vi "capstone2.vi"() -> ()   [LabVIEW 2016]
uses:
  <instrlib>/Dynamixel Motor/Public/Motor Operation/Low Level/Baud Setting.ctl
  <vilib>/myRIO/Instrument Drivers/Onboard IO/DIO/typedefs/DIO Reference.ctl
  <vilib>/myRIO/Common/Instrument Driver Framework/Utilities/typedefs/myRIO Generic Hardware Reference.ctl
  <vilib>/myRIO/Common/Instrument Driver Framework/Utilities/typedefs/Hardware Version Enum.ctl
  <vilib>/myRIO/Common/Instrument Driver Framework/Utilities/typedefs/myRIO v1.0 Reference.ctl
  <vilib>/myRIO/Common/Instrument Driver Framework/Utilities/typedefs/Generic FPGA Reference.ctl
  <vilib>/myRIO/Common/Instrument Driver Framework/myRIO v1.0/DIO/typedefs/DIO Channels List.ctl
  <vilib>/myRIO/Common/Instrument Driver Framework/myRIO v1.0/DIO/typedefs/DIO Channels Enum.ctl
  <vilib>/userdefined/High Color/nirio_resource_hc.ctl
  <vilib>/myRIO/Common/Instrument Driver Framework/Utilities/vis/Is FPGA Ref Available.vi
  <vilib>/myRIO/Common/Instrument Driver Framework/myRIO v1.0/DIO/vis/myRIO v1.1 Open DIO.vi
  <vilib>/myRIO/Instrument Drivers/Onboard IO/DIO/vis/Write.vi
  <vilib>/myRIO/Common/Instrument Driver Framework/Utilities/vis/Validate Channels.vi
  <vilib>/myRIO/Common/Instrument Driver Framework/myRIO v1.0/DIO/vis/myRIO v1.0 Reserve DIO.vi
  <vilib>/myRIO/Common/Instrument Driver Framework/myRIO v1.0/UART/vis/myRIO v1.0 Close UART.vi
  <vilib>/myRIO/Common/Instrument Driver Framework/myRIO v1.0/Resource Manager/vis/myRIO v1.0 Reserve Channel List.vi
  <vilib>/myRIO/Common/Instrument Driver Framework/myRIO v1.0/DIO/vis/myRIO v1.0 Build MUX Configuration DIO.vi
  <vilib>/myRIO/Common/Instrument Driver Framework/myRIO v1.0/Resource Manager/vis/myRIO v1.0 Reserve Channel.vi
  <vilib>/myRIO/Common/Instrument Driver Framework/myRIO v1.0/Resource Manager/vis/myRIO v1.0 Unreserve Channel.vi
  <vilib>/myRIO/Common/Instrument Driver Framework/myRIO v1.0/Resource Manager/vis/myRIO v1.0 Create Configuration List.vi
  <vilib>/myRIO/Common/Instrument Driver Framework/myRIO v1.0/Resource Manager/vis/myRIO v1.0 Build Mutex Name.vi
  <vilib>/Utility/VariantDataType/GetNumericInfo.vi
  <vilib>/Utility/error.llb/Error Cluster From Error Code.vi
  <vilib>/myRIO/Common/Instrument Driver Framework/myRIO v1.0/myRIO v1.1 Open.vi
  <vilib>/myRIO/Common/Instrument Driver Framework/Utilities/vis/IO Manager.vi
  <vilib>/myRIO/Common/Instrument Driver Framework/Utilities/vis/Configuration Manager.vi
  <vilib>/myRIO/Common/Instrument Driver Framework/myRIO v1.0/Resource Manager/vis/myRIO v1.0 Configure IO.vi
  <vilib>/myRIO/Common/Instrument Driver Framework/myRIO v1.0/myRIO v1.0 Close.vi
  <vilib>/myRIO/Common/Instrument Driver Framework/myRIO v1.0/DIO/vis/myRIO v1.0 Write DIO.vi
  <vilib>/myRIO/Common/Instrument Driver Framework/Utilities/vis/FPGA Ref Manager.vi
  <vilib>/myRIO/Common/Instrument Driver Framework/myRIO v1.0/myRIO v1.0 Reset FPGA.vi
  <vilib>/myRIO/Common/Instrument Driver Framework/myRIO v1.0/IRQ/vis/myRIO v1.0 IRQ Info FGV.vi
  <vilib>/myRIO/Common/Instrument Driver Framework/myRIO v1.0/IRQ/vis/myRIO v1.0 Timer IRQ Info FGV.vi
  <vilib>/myRIO/Common/Instrument Driver Framework/myRIO v1.0/IRQ/vis/myRIO v1.0 ISR Agent.vi
  <vilib>/myRIO/Express VI/Onboard Devices/LED/LED Express VI.xnode
  <vilib>/myRIO/Instrument Drivers/Onboard IO/DIO/vis/myRIO DIO Open.xnode
  <instrlib>/Dynamixel Motor/Dynamixel Motor.lvlib
  <vilib>/myRIO/Instrument Drivers/Onboard IO/DIO/DIO.lvlib
  <vilib>/myRIO/Instrument Drivers/Utilities/Utilities.lvlib
panel:
  in  "main stop":bool
  out "RT TCP Loop time":u32
  out "value":T1
  out "TCP Read data":string
  in  "정지":bool
  out "error out":errorcluster
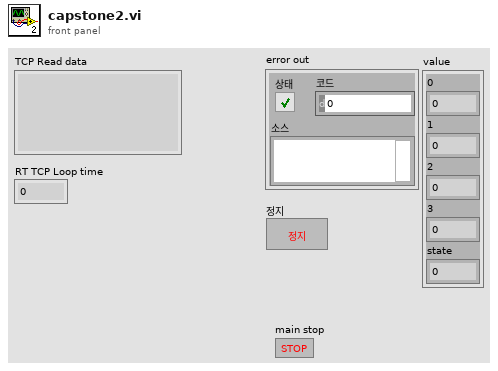
[diagram p1: front panel]
types:
  T1 = cluster{"0":sgl, "1":sgl, "2":sgl, "3":sgl, "state":sgl}
  T2 = typedef "DIO.lvlib/DIO Reference.ctl" = cluster{"myRIO Reference":T3, "DIO Channels List":T7}
  T3 = typedef "myRIO Generic Hardware Reference.ctl" = cluster{"myRIO Model":T4, "myRIO Hardware Reference":T5}
  T4 = typedef "Hardware Version Enum.ctl" = enum16{"Unknown", "myRIO-1900", "myRIO-1950", "roboRIO", "NI ELVIS RIO CM"}
  T5 = typedef "myRIO v1.0 Reference.ctl" = cluster{"Generic FPGA Reference":T6, "Allow multiple opens":bool}
  T6 = typedef "Generic FPGA Reference.ctl" = refnum<k20>
  T7 = typedef "DIO Channels List.ctl" = T8[]
  T8 = typedef "DIO Channels Enum.ctl" = enum16{"Not Connected", "C/DIO0", "C/DIO1", "C/DIO2", "C/DIO3", "C/DIO4", "C/DIO5", "C/DIO6", "C/DIO7", "A/DIO0", "A/DIO1", "A/DIO2", "A/DIO3", "A/DIO4", "A/DIO5", "A/DIO6", "A/DIO7", "A/DIO8", "A/DIO9", "A/DIO10", "A/DIO11", "A/DIO12", "A/DIO13", "A/DIO14", "A/DIO15", "B/DIO0", "B/DIO1", "B/DIO2", "B/DIO3", "B/DIO4", "B/DIO5", "B/DIO6", "B/DIO7", "B/DIO8", "B/DIO9", "B/DIO10", "B/DIO11", "B/DIO12", "B/DIO13", "B/DIO14", "B/DIO15", "LED0", "LED1", "LED2", "LED3", "Button0", "DIO/DIO0", "DIO/DIO1", "DIO/DIO2", "DIO/DIO3", "DIO/DIO4", "DIO/DIO5", "DIO/DIO6", "DIO/DIO7", "DIO/DIO8", "DIO/DIO9", "SPI/CS0", "SPI/CS1", "SPI/CS2", "SPI/CS3", "LED RADIO (Green)", "LED RADIO (Red)", "LED COMM (Green)", "LED COMM (Red)", "LED MODE (Green)", "LED MODE (Red)"}
  T9 = typedef "nirio_resource_hc.ctl" = tag
  T10 = cluster{"0":sgl, "1":sgl, "2":sgl, "3":sgl, "state":i32}
  T11 = typedef "Dynamixel Motor.lvlib/Baud Setting.ctl" = u8
  T12 = enum16{"big-endian, network order", "native, host order", "little-endian"}
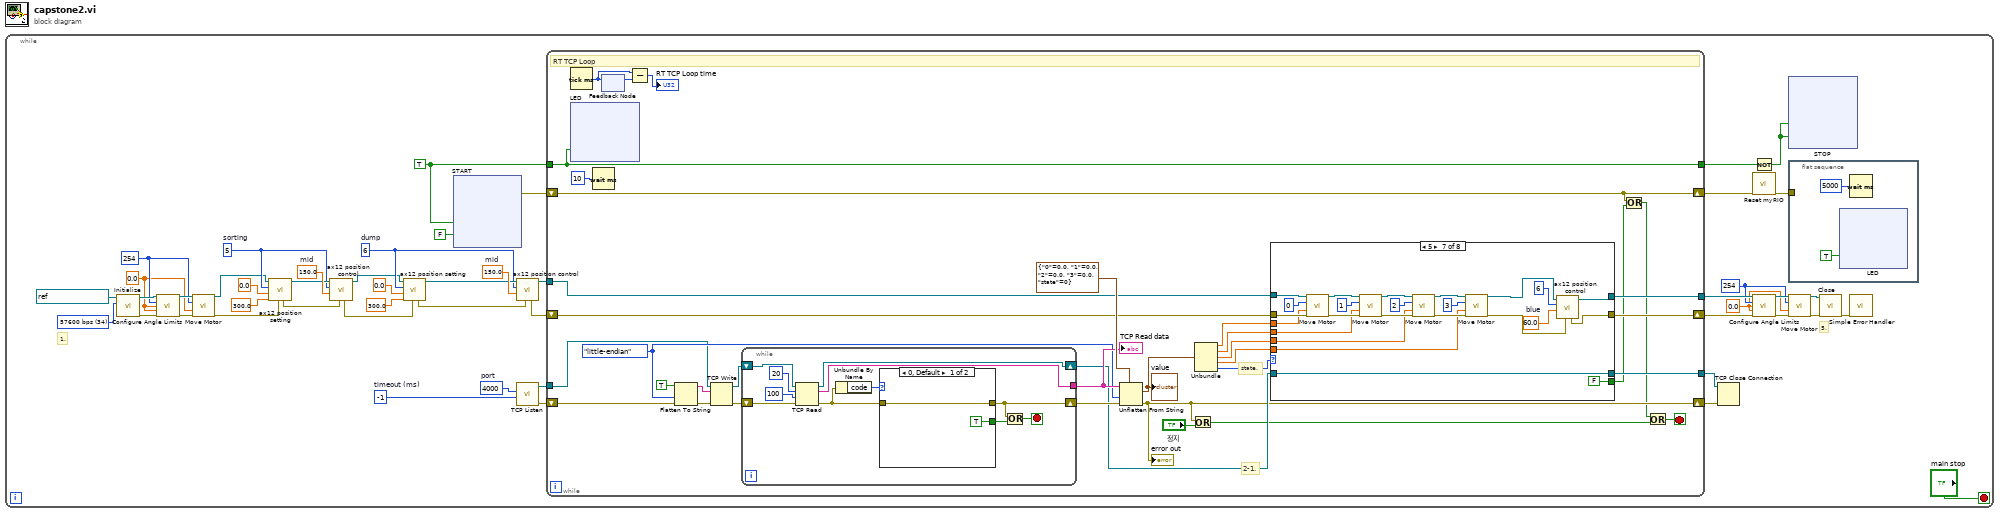
[diagram p0: block diagram]
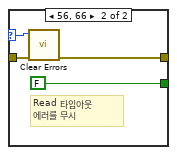
[diagram p2: hidden frame]
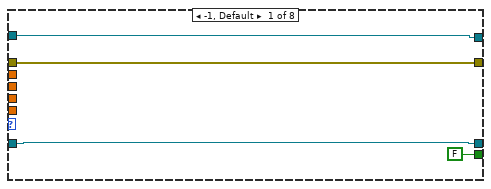
[diagram p3: hidden frame]
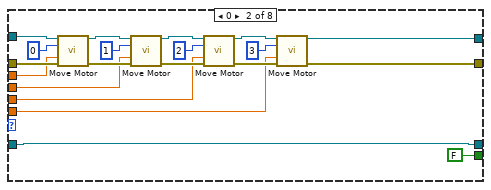
[diagram p4: hidden frame]
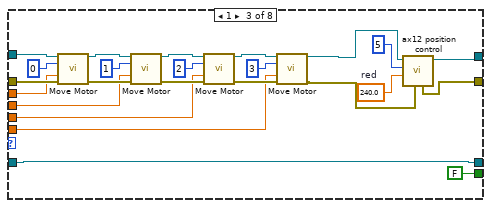
[diagram p5: hidden frame]
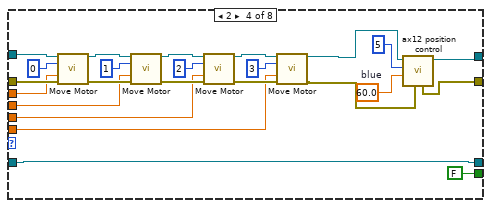
[diagram p6: hidden frame]
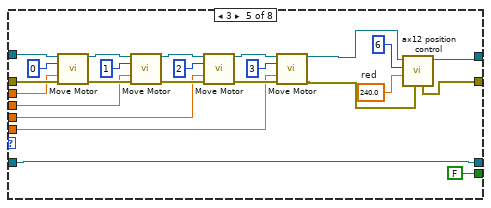
[diagram p7: hidden frame]
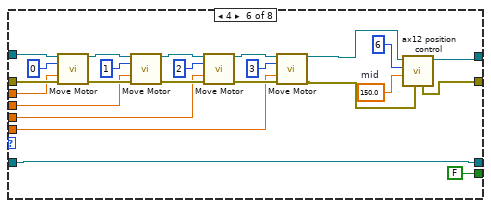
[diagram p8: hidden frame]
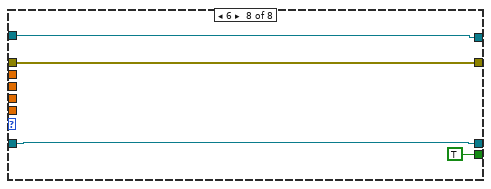
[diagram p9: hidden frame]
diagram:
  n1 = while {
    stop <- "main stop" stop-if-true
    w8 = 150.0  # mid
    w6 = 5  # sorting
    w16 = 150.0  # mid
    w14 = 6  # dump
    w44 = T11 34 items=["1,000,000 bps"=1, "500,000 bps"=3, "400,000 bps"=4, "250,000 bps"=7, "200,000 bps"=9, "115200 bps"=16, "57600 bps"=34, "19200 bps"=103, "9600 bps"=207] ("Baud rate (57600 bps)")
    w34 = TRUE
    w24 = 0.0 ("Goal Speed (RPM)")
    w25 = u8 254 ("Motor ID (0)")
    w36 = u8 254 ("Motor ID (0)")
    w35 = 0.0 ("Clockwise Angle Limit (0 deg)")
    w48 = u16 4000  # port
    w49 = -1  # timeout (ms)
    # "5."
    # "1."
    n2 = call <instrlib>:"Initialize.vi"("Baud rate (57600 bps)"=w44, "VISA resource name"=refnum<visa-resource-name> "ASRL3::INSTR") -> ("error out"=w40:errorcluster, "VISA resource name out"=w39:refnum<visa-resource-name>)  [unwired: 8 in]
    n3 = call <instrlib>:"Configure Angle Limits.vi"("VISA resource name"=w39, "Motor ID (0)"=w36, "Clockwise Angle Limit (0 deg)"=w35, "Counter-Clockwise Angle Limit (300 deg)"=w35, "error in (no error)"=w40) -> ("VISA resource name out"=w38:refnum<visa-resource-name>, "error out"=w37:errorcluster)  [unwired: 9 in]
    n4 = call <instrlib>:"Move Motor.vi"("VISA resource name"=w38, "Motor ID (0)"=w36, "Goal Speed (RPM)"=w35, "error in (no error)"=w37) -> ("VISA resource name out"=w4:refnum<visa-resource-name>, "error out"=w3:errorcluster)  [unwired: 10 in]
    n5 = call "ax12 position setting.vi"("error in (no error)"=w3, "Counter-Clockwise Angle Limit (300 deg)"=300.0 ("Clockwise Angle Limit (0 deg)"), "Clockwise Angle Limit (0 deg)"=0.0, "Motor ID (0)"=w6, "VISA resource name"=w4) -> ("VISA resource name out"=w7:refnum<visa-resource-name>, "error out"=w5:errorcluster)  [unwired: 5 in]
    n6 = call "ax12 position control.vi"("error in (no error)"=w5, "Goal Position (180 deg)"=w8, "Motor ID (0)"=w6, "VISA resource name"=w7) -> ("VISA resource name out"=w1:refnum<visa-resource-name>, "error out"=w2:errorcluster)  [unwired: 6 in]
    n7 = call "ax12 position setting.vi"("error in (no error)"=w2, "Counter-Clockwise Angle Limit (300 deg)"=300.0 ("Clockwise Angle Limit (0 deg)"), "Clockwise Angle Limit (0 deg)"=0.0, "Motor ID (0)"=w14, "VISA resource name"=w1) -> ("VISA resource name out"=w15:refnum<visa-resource-name>, "error out"=w11:errorcluster)  [unwired: 5 in]
    n8 = xnode "START"("LED0"=w34, "LED3"=FALSE) -> ("error out"=w20:errorcluster)  [unwired: 1 in]
    n9 = call "ax12 position control.vi"("error in (no error)"=w11, "Goal Position (180 deg)"=w16, "Motor ID (0)"=w14, "VISA resource name"=w15) -> ("VISA resource name out"=w13:refnum<visa-resource-name>, "error out"=w12:errorcluster)  [unwired: 6 in]
    n10 = call <vilib>:"TCP Listen.vi"("timeout ms (wait forever: -1)"=w49, "port"=w48) -> ("error out"=w45:errorcluster, "connection ID"=w31:refnum<k5>)  [unwired: 5 in, 3 out]
    n11 = while {
      tunnel: w31 -> [w169]
      tunnel: [w174] -> w47
      shift-right: [w165] -> w46
      shift-left: w45 -> [w166]
      shift-right: [w181] -> w29
      shift-left: w12 -> [w180]
      tunnel: w34 -> [w189]
      tunnel: [w189] -> w42
      tunnel: [w182] -> w27
      shift-right: [w160] -> w19
      shift-left: w20 -> [w160]
      tunnel: w13 -> [w162]
      stop <- w163 stop-if-true
      w170 = T12."little-endian" ("byte order (0:big-endian, network order)")
      # "state."
      # "2-1."
      # "RT TCP Loop"
      n12 = Tick Count (ms)() -> (millisecond timer value=w178:u32)
      n13 = xnode "LED"("LED1"=w189) -> ()  [unwired: 1 in, 1 out]
      n14 = Wait (ms)(milliseconds to wait=u32 10 ("대기 시간 (ms)")) -> ()  [unwired: 1 out]
      n15 = feedback #1() -> (w179:u32)  [unwired: 1 in]
      n16 = feedback-in #1(w178) -> ()
      n17 = Subtract(x=w178, y=w179) -> (x-y=→"RT TCP Loop time":u32)
      n18 = Flatten To String(anything=TRUE, byte order (0:big-endian, network order)=w170, error in (no error)=w166) -> (data string=w173:string, error out=w172:errorcluster)  [unwired: 1 in, 1 out]
      n19 = TCP Write(connection ID=w169, data in=w173, error in (no error)=w172) -> (connection ID out=w168:refnum<k5>, error out=w167:errorcluster)  [unwired: 1 in, 1 out]
      n20 = while {
        tunnel: [w202] -> w191
        shift-right: [w201] -> w175
        shift-left: w168 -> [w200]
        shift-right: [w196] -> w190
        shift-left: w167 -> [w199]
        stop <- w194 stop-if-true
        n21 = TCP Read(connection ID=w200, bytes to read=20 ("읽을 바이트"), error in (no error)=w199, 9:100 ("타임아웃 ms (25000)")) -> (connection ID out=w201:refnum<k5>, data out=w202:string, error out=w197:errorcluster)  [unwired: 1 in]
        n22 = Unbundle By Name(w197) -> ("code"=w198:i32)
        n23 = case shown="0, Default" w198 {
          selector: w198 -> [_ w209]
          tunnel: [w206 w208] -> w196
          tunnel: w197 -> [w206 w210]
          tunnel: [TRUE FALSE] -> w195
          frame 0, Default {
          }
          frame 56, 66 {
            # "Read 타임아웃\n에러를 무시"
            n24 = call <vilib>:"Clear Errors.vi"("error in (no error)"=w210, "specific error code to clear (0: all)"=w209) -> ("error out"=w208:errorcluster)  [unwired: 4 in, 1 out]
          }
        }
        n25 = Or(x=w196, y=w195) -> (x .or. y?=w194:bool)
      }
      "TCP Read data" <- w191
      n26 = Unflatten From String(type=T10 {"0"=0.0, "1"=0.0, "2"=0.0, "3"=0.0, "state"=0}, binary string=w191, byte order (0:big-endian, network order)=w170, error in (no error)=w190) -> (value=w188:T10, error out=w165:errorcluster)  [unwired: 1 in, 1 out]
      "error out" <- w165
      "value" <- w188
      n27 = Or(x=w165, y="정지") -> (x .or. y?=w159:bool)
      n28 = Unbundle(w188) -> ("0"=w187:sgl, "1"=w185:sgl, "2"=w186:sgl, "3"=w184:sgl, "state"=w183:i32)
      n29 = case shown="5" w183 {
        tunnel: w187 -> [_ w219 w245 w269 w293 w317 w341 _]
        tunnel: w185 -> [_ w218 w244 w268 w292 w316 w340 _]
        tunnel: w186 -> [_ w217 w243 w267 w291 w315 w339 _]
        tunnel: w184 -> [_ w216 w242 w266 w290 w314 w338 _]
        tunnel: [w214 w225 w236 w260 w284 w308 w332 w355] -> w182
        tunnel: [w213 w226 w235 w259 w283 w307 w331 w356] -> w181
        tunnel: w180 -> [w213 w221 w247 w271 w295 w319 w343 w356]
        tunnel: w162 -> [w214 w220 w246 w270 w294 w318 w342 w355]
        tunnel: w175 -> [w212 w223 w249 w273 w297 w321 w345 w358]
        tunnel: [w212 w223 w249 w273 w297 w321 w345 w358] -> w174
        tunnel: [FALSE FALSE FALSE FALSE FALSE FALSE FALSE TRUE] -> w161
        frame -1, Default {
        }
        frame 0 {
          n30 = call <instrlib>:"Move Motor.vi"("VISA resource name"=w220, "Motor ID (0)"=0, "Goal Speed (RPM)"=w219, "error in (no error)"=w221) -> ("VISA resource name out"=w229:refnum<visa-resource-name>, "error out"=w230:errorcluster)  [unwired: 10 in]
          n31 = call <instrlib>:"Move Motor.vi"("VISA resource name"=w229, "Motor ID (0)"=1, "Goal Speed (RPM)"=w218, "error in (no error)"=w230) -> ("VISA resource name out"=w231:refnum<visa-resource-name>, "error out"=w233:errorcluster)  [unwired: 10 in]
          n32 = call <instrlib>:"Move Motor.vi"("VISA resource name"=w231, "Motor ID (0)"=2, "Goal Speed (RPM)"=w217, "error in (no error)"=w233) -> ("VISA resource name out"=w232:refnum<visa-resource-name>, "error out"=w234:errorcluster)  [unwired: 10 in]
          n33 = call <instrlib>:"Move Motor.vi"("VISA resource name"=w232, "Motor ID (0)"=u8 3, "Goal Speed (RPM)"=w216, "error in (no error)"=w234) -> ("VISA resource name out"=w225:refnum<visa-resource-name>, "error out"=w226:errorcluster)  [unwired: 10 in]
        }
        frame 1 {
          w240 = 240.0  # red
          n34 = call <instrlib>:"Move Motor.vi"("VISA resource name"=w246, "Motor ID (0)"=0, "Goal Speed (RPM)"=w245, "error in (no error)"=w247) -> ("VISA resource name out"=w253:refnum<visa-resource-name>, "error out"=w254:errorcluster)  [unwired: 10 in]
          n35 = call <instrlib>:"Move Motor.vi"("VISA resource name"=w253, "Motor ID (0)"=1, "Goal Speed (RPM)"=w244, "error in (no error)"=w254) -> ("VISA resource name out"=w255:refnum<visa-resource-name>, "error out"=w257:errorcluster)  [unwired: 10 in]
          n36 = call <instrlib>:"Move Motor.vi"("VISA resource name"=w255, "Motor ID (0)"=2, "Goal Speed (RPM)"=w243, "error in (no error)"=w257) -> ("VISA resource name out"=w256:refnum<visa-resource-name>, "error out"=w258:errorcluster)  [unwired: 10 in]
          n37 = call <instrlib>:"Move Motor.vi"("VISA resource name"=w256, "Motor ID (0)"=u8 3, "Goal Speed (RPM)"=w242, "error in (no error)"=w258) -> ("VISA resource name out"=w238:refnum<visa-resource-name>, "error out"=w237:errorcluster)  [unwired: 10 in]
          n38 = call "ax12 position control.vi"("error in (no error)"=w237, "Goal Position (180 deg)"=w240, "Motor ID (0)"=u8 5, "VISA resource name"=w238) -> ("VISA resource name out"=w236:refnum<visa-resource-name>, "error out"=w235:errorcluster)  [unwired: 6 in]
        }
        frame 2 {
          w264 = 60.0  # blue
          n39 = call <instrlib>:"Move Motor.vi"("VISA resource name"=w270, "Motor ID (0)"=0, "Goal Speed (RPM)"=w269, "error in (no error)"=w271) -> ("VISA resource name out"=w277:refnum<visa-resource-name>, "error out"=w278:errorcluster)  [unwired: 10 in]
          n40 = call <instrlib>:"Move Motor.vi"("VISA resource name"=w277, "Motor ID (0)"=1, "Goal Speed (RPM)"=w268, "error in (no error)"=w278) -> ("VISA resource name out"=w279:refnum<visa-resource-name>, "error out"=w281:errorcluster)  [unwired: 10 in]
          n41 = call <instrlib>:"Move Motor.vi"("VISA resource name"=w279, "Motor ID (0)"=2, "Goal Speed (RPM)"=w267, "error in (no error)"=w281) -> ("VISA resource name out"=w280:refnum<visa-resource-name>, "error out"=w282:errorcluster)  [unwired: 10 in]
          n42 = call <instrlib>:"Move Motor.vi"("VISA resource name"=w280, "Motor ID (0)"=u8 3, "Goal Speed (RPM)"=w266, "error in (no error)"=w282) -> ("VISA resource name out"=w262:refnum<visa-resource-name>, "error out"=w261:errorcluster)  [unwired: 10 in]
          n43 = call "ax12 position control.vi"("error in (no error)"=w261, "Goal Position (180 deg)"=w264, "Motor ID (0)"=u8 5, "VISA resource name"=w262) -> ("VISA resource name out"=w260:refnum<visa-resource-name>, "error out"=w259:errorcluster)  [unwired: 6 in]
        }
        frame 3 {
          w288 = 240.0  # red
          n44 = call <instrlib>:"Move Motor.vi"("VISA resource name"=w294, "Motor ID (0)"=0, "Goal Speed (RPM)"=w293, "error in (no error)"=w295) -> ("VISA resource name out"=w301:refnum<visa-resource-name>, "error out"=w302:errorcluster)  [unwired: 10 in]
          n45 = call <instrlib>:"Move Motor.vi"("VISA resource name"=w301, "Motor ID (0)"=1, "Goal Speed (RPM)"=w292, "error in (no error)"=w302) -> ("VISA resource name out"=w303:refnum<visa-resource-name>, "error out"=w305:errorcluster)  [unwired: 10 in]
          n46 = call <instrlib>:"Move Motor.vi"("VISA resource name"=w303, "Motor ID (0)"=2, "Goal Speed (RPM)"=w291, "error in (no error)"=w305) -> ("VISA resource name out"=w304:refnum<visa-resource-name>, "error out"=w306:errorcluster)  [unwired: 10 in]
          n47 = call <instrlib>:"Move Motor.vi"("VISA resource name"=w304, "Motor ID (0)"=u8 3, "Goal Speed (RPM)"=w290, "error in (no error)"=w306) -> ("VISA resource name out"=w286:refnum<visa-resource-name>, "error out"=w285:errorcluster)  [unwired: 10 in]
          n48 = call "ax12 position control.vi"("error in (no error)"=w285, "Goal Position (180 deg)"=w288, "Motor ID (0)"=u8 6, "VISA resource name"=w286) -> ("VISA resource name out"=w284:refnum<visa-resource-name>, "error out"=w283:errorcluster)  [unwired: 6 in]
        }
        frame 4 {
          w312 = 150.0  # mid
          n49 = call <instrlib>:"Move Motor.vi"("VISA resource name"=w318, "Motor ID (0)"=0, "Goal Speed (RPM)"=w317, "error in (no error)"=w319) -> ("VISA resource name out"=w325:refnum<visa-resource-name>, "error out"=w326:errorcluster)  [unwired: 10 in]
          n50 = call <instrlib>:"Move Motor.vi"("VISA resource name"=w325, "Motor ID (0)"=1, "Goal Speed (RPM)"=w316, "error in (no error)"=w326) -> ("VISA resource name out"=w327:refnum<visa-resource-name>, "error out"=w329:errorcluster)  [unwired: 10 in]
          n51 = call <instrlib>:"Move Motor.vi"("VISA resource name"=w327, "Motor ID (0)"=2, "Goal Speed (RPM)"=w315, "error in (no error)"=w329) -> ("VISA resource name out"=w328:refnum<visa-resource-name>, "error out"=w330:errorcluster)  [unwired: 10 in]
          n52 = call <instrlib>:"Move Motor.vi"("VISA resource name"=w328, "Motor ID (0)"=u8 3, "Goal Speed (RPM)"=w314, "error in (no error)"=w330) -> ("VISA resource name out"=w310:refnum<visa-resource-name>, "error out"=w309:errorcluster)  [unwired: 10 in]
          n53 = call "ax12 position control.vi"("error in (no error)"=w309, "Goal Position (180 deg)"=w312, "Motor ID (0)"=u8 6, "VISA resource name"=w310) -> ("VISA resource name out"=w308:refnum<visa-resource-name>, "error out"=w307:errorcluster)  [unwired: 6 in]
        }
        frame 5 {
          w336 = 60.0  # blue
          n54 = call <instrlib>:"Move Motor.vi"("VISA resource name"=w342, "Motor ID (0)"=0, "Goal Speed (RPM)"=w341, "error in (no error)"=w343) -> ("VISA resource name out"=w349:refnum<visa-resource-name>, "error out"=w350:errorcluster)  [unwired: 10 in]
          n55 = call <instrlib>:"Move Motor.vi"("VISA resource name"=w349, "Motor ID (0)"=1, "Goal Speed (RPM)"=w340, "error in (no error)"=w350) -> ("VISA resource name out"=w351:refnum<visa-resource-name>, "error out"=w353:errorcluster)  [unwired: 10 in]
          n56 = call <instrlib>:"Move Motor.vi"("VISA resource name"=w351, "Motor ID (0)"=2, "Goal Speed (RPM)"=w339, "error in (no error)"=w353) -> ("VISA resource name out"=w352:refnum<visa-resource-name>, "error out"=w354:errorcluster)  [unwired: 10 in]
          n57 = call <instrlib>:"Move Motor.vi"("VISA resource name"=w352, "Motor ID (0)"=u8 3, "Goal Speed (RPM)"=w338, "error in (no error)"=w354) -> ("VISA resource name out"=w334:refnum<visa-resource-name>, "error out"=w333:errorcluster)  [unwired: 10 in]
          n58 = call "ax12 position control.vi"("error in (no error)"=w333, "Goal Position (180 deg)"=w336, "Motor ID (0)"=u8 6, "VISA resource name"=w334) -> ("VISA resource name out"=w332:refnum<visa-resource-name>, "error out"=w331:errorcluster)  [unwired: 6 in]
        }
        frame 6 {
        }
      }
      n59 = Or(x=w160, y=w161) -> (x .or. y?=w164:bool)
      n60 = Or(x=w164, y=w159) -> (x .or. y?=w163:bool)
    }
    n61 = TCP Close Connection(connection ID=w47, error in (no error)=w46) -> ()  [unwired: 3 out]
    n62 = Not(x=w42) -> (.not. x?=w41:bool)
    n63 = call <vilib>:"Reset myRIO.vi"("error in (no error)"=w19) -> ("error out"=w23:errorcluster)  [unwired: 10 in]
    n64 = call <instrlib>:"Configure Angle Limits.vi"("VISA resource name"=w27, "Motor ID (0)"=w25, "Clockwise Angle Limit (0 deg)"=w24, "Counter-Clockwise Angle Limit (300 deg)"=w24, "error in (no error)"=w29) -> ("VISA resource name out"=w26:refnum<visa-resource-name>, "error out"=w28:errorcluster)  [unwired: 9 in]
    n65 = xnode "STOP"("LED0"=w41, "LED1"=w41) -> ()  [unwired: 1 in, 1 out]
    n66 = flat-sequence {
      tunnel: w23 -> [_]
      frame #0 {
        n67 = xnode "LED"("LED3"=TRUE) -> ()  [unwired: 1 in, 1 out]
        n68 = Wait (ms)(milliseconds to wait=5000) -> ()  [unwired: 1 out]
      }
    }
    n69 = call <instrlib>:"Move Motor.vi"("VISA resource name"=w26, "Motor ID (0)"=w25, "Goal Speed (RPM)"=w24, "error in (no error)"=w28) -> ("VISA resource name out"=w33:refnum<visa-resource-name>, "error out"=w32:errorcluster)  [unwired: 10 in]
    n70 = call <instrlib>:"Close.vi"("error in (no error)"=w32, "VISA resource name"=w33) -> ("error out"=w30:errorcluster)  [unwired: 9 in]
    n71 = call <vilib>:"Simple Error Handler.vi"("error in (no error)"=w30) -> ()  [unwired: 4 in, 5 out]
  }
